vi "02_WhyVIMs.vi"() -> ()   [LabVIEW 2017]
uses:
  2f5f1c39-255c-4448-b063-fb8cf7db9d41.vi
panel:
  out "millisecond timer value":u32
  in  "milliseconds to wait":u32
  out "value out":variant
  in  "value in":variant
  out "Numeric Indicator":dbl
  in  "Numeric Control":dbl
  out "String Indicator":string
  in  "String Control":string
  # "So why VIMs?"
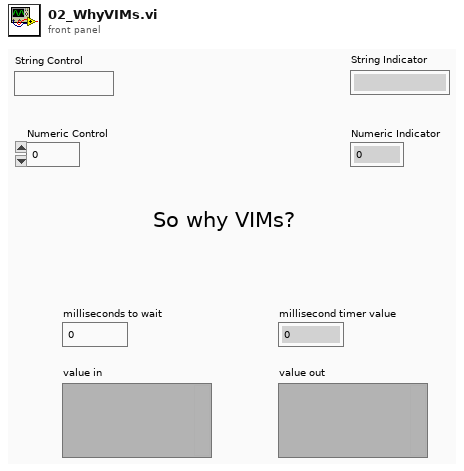
[diagram p1: front panel]
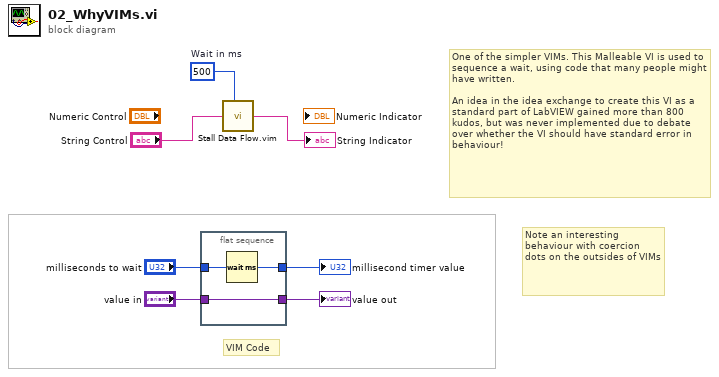
[diagram p0: block diagram]
diagram:
  w1 = 500  # Wait in ms
  # "Note an interesting behaviour with coercion dots on the outsides of VIMs"
  # "One of the simpler VIMs. This Malleable VI is used to sequence a wait, using code that many people might have written.\n\nAn idea in the idea exchange to create this VI as a standard part of LabVIEW gained more than 800 kudos, but was never implemented due to debate over whether the VI should have standard error in behaviour!"
  # "VIM Code"
  n1 = flat-sequence {
    tunnel: "milliseconds to wait" -> [w10]
    tunnel: [w9] -> w4
    tunnel: [w8] -> w3
    tunnel: "value in" -> [w8]
    frame #0 {
      n2 = Wait (ms)(milliseconds to wait=w10) -> (millisecond timer value=w9:u32)
    }
  }
  n3 = call "Stall Data Flow.vim"("value in"="String Control", "milliseconds to wait"=w1) -> ("value out"=→"String Indicator":string)  [unwired: 1 out]
  "value out" <- w3
  "millisecond timer value" <- w4
